vi "Calculate Persistence Path.vi"(0 "User Manager Model in":refnum<class "User Manager Model.lvclass">, 11 "error in (no error)":errorcluster) -> (4 "User Manager Model out":refnum<class "User Manager Model.lvclass">, 15 "error out":errorcluster)   [LabVIEW 2017, in "User Manager Model.lvlib" / "User Manager Model.lvclass"]
uses:
  <vilib>/gpm_packages/@cs/User Manager App/User Manager Model/User Manager Model/User Manager Model.lvclass
  <vilib>/gpm_packages/@cs/User Manager App/User Manager Model/User Manager Model/User Manager Model.lvclass/User Manager Model.ctl
  <vilib>/gpm_packages/@cs/User Manager App/User Manager Model/User Manager Model/Accessors/Write Persistence Path.vi
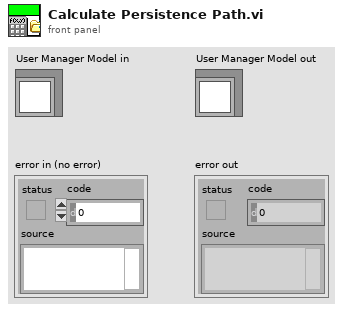
[diagram p1: front panel]
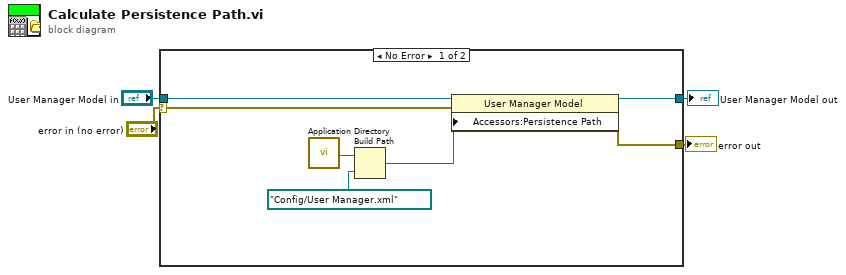
[diagram p0: block diagram]
diagram:
  n1 = case shown="No Error" "error in (no error)" {
    selector: "error in (no error)" -> [w6 w13]
    tunnel: [w7 w13] -> w3
    tunnel: [w9 w12] -> w1
    tunnel: "User Manager Model in" -> [w11 w12]
    frame No Error {
      n2 = call <vilib>:"Application Directory.vi"() -> ("Application Directory"=w5:path)
      n3 = Build Path(base path=w5, name or relative path=path "Config/User Manager.xml") -> (appended path=w8:path)
      n4 = property class="User Manager Model"(reference=w11, error in=w6, "Accessors:Persistence Path"=w8) -> (reference out=w9:refnum<class "User Manager Model.lvclass">, error out=w7:errorcluster)
    }
    frame Error {
    }
  }
  "error out" <- w3
  "User Manager Model out" <- w1
